vi "Parse Summary String.vi"(11 "Summary String":string) -> (3 "Test Header":T1={"name"="", "tests"=-1, "failures"=-1, "errors"=-1, "time"=-1.0, "disabled"=-1, "skipped"=-1, "skips"=-1, "timestamp"=-1.0, "hostname"="", "id"="", "package"="", "assertions"=-1, "file"="", "skip"="", "log"="", "url"=""})   [LabVIEW 2014, in "VI Tester Parsing.lvlib"]
uses:
  VI Tester Parsing.lvlib
  <vilib>/ni/JUnit Results API/Controls/Test Suite Attribute Values.ctl
  <vilib>/ni/JUnit Results API/JUnit API.lvlib
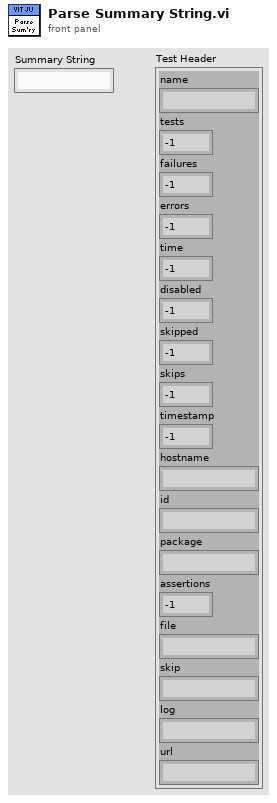
[diagram p1: front panel]
types:
  T1 = typedef "JUnit API.lvlib/Test Suite Attribute Values.ctl" = cluster{"name":string, "tests":i32, "failures":i32, "errors":i32, "time":dbl, "disabled":i32, "skipped":i32, "skips":i32, "timestamp":dbl, "hostname":string, "id":string, "package":string, "assertions":i32, "file":string, "skip":string, "log":string, "url":string}
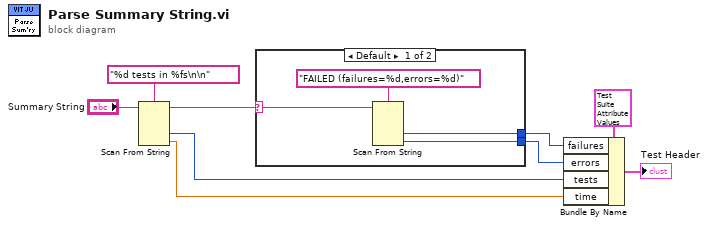
[diagram p0: block diagram]
diagram:
  n1 = Scan From String(format string="%d tests in %fs\n\n", input string="Summary String") -> (remaining string=w6:string, output 1=w1:i32, output 2=w8:dbl)  [unwired: 4 in, 2 out]
  n2 = case shown="Default" w6 {
    selector: w6 -> [w12 _]
    tunnel: [w11 _] -> w3
    tunnel: [w10 _] -> w2
    frame Default {
      n3 = Scan From String(format string="FAILED (failures=%d,errors=%d)", input string=w12) -> (output 1=w11:i32, output 2=w10:i32)  [unwired: 4 in, 3 out]
    }
    frame "OK" {
    }
  }
  n4 = Bundle By Name(cluster=T1 {"name"="", "tests"=-1, "failures"=-1, "errors"=-1, "time"=-1.0, "disabled"=-1, "skipped"=-1, "skips"=-1, "timestamp"=-1.0, "hostname"="", "id"="", "package"="", "assertions"=-1, "file"="", "skip"="", "log"="", "url"=""} ("Test Suites Atrributes"), "failures"=w3, "errors"=w2, "tests"=w1, "time"=w8) -> (→"Test Header":T1)
